vi "VISA Write and Read.vi"(6 "Delay":u32=50, 7 "Checksum":T1, 8 "error in (no error)":errorcluster, 10 "Command":string, 11 "VISA In":refnum<visa-resource-name>) -> (0 "error out":errorcluster, 2 "Response":string, 3 "VISA Out":refnum<visa-resource-name>)   [LabVIEW 2014, in "VISA.lvlib"]
uses:
  VISA.lvlib
  Checksum.ctl
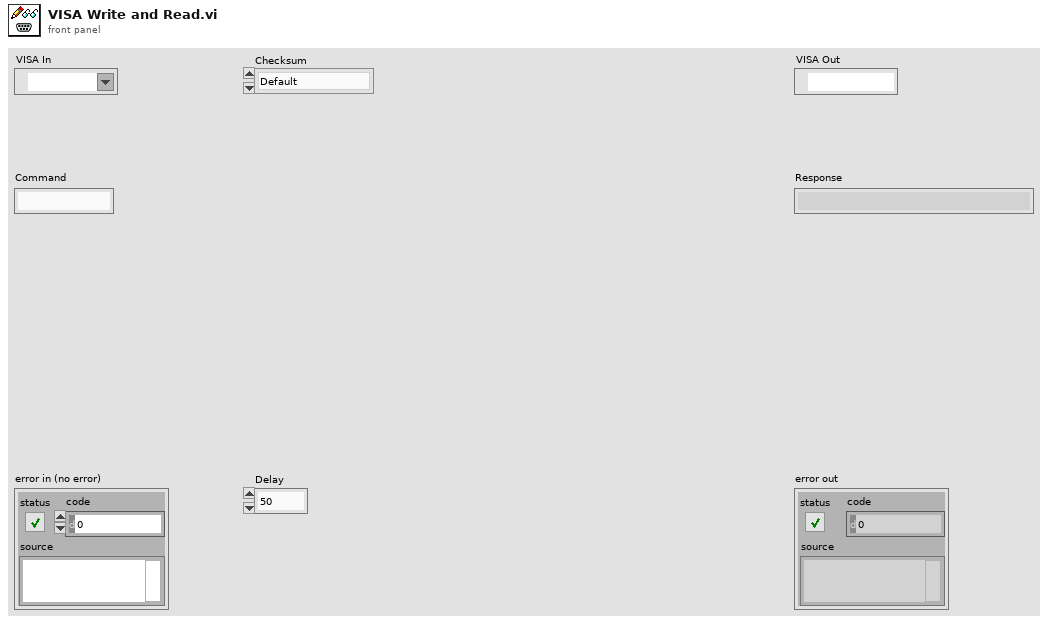
[diagram p1: front panel]
types:
  T1 = typedef "VISA.lvlib/Checksum.ctl" = enum16{"Default", "CRC"}
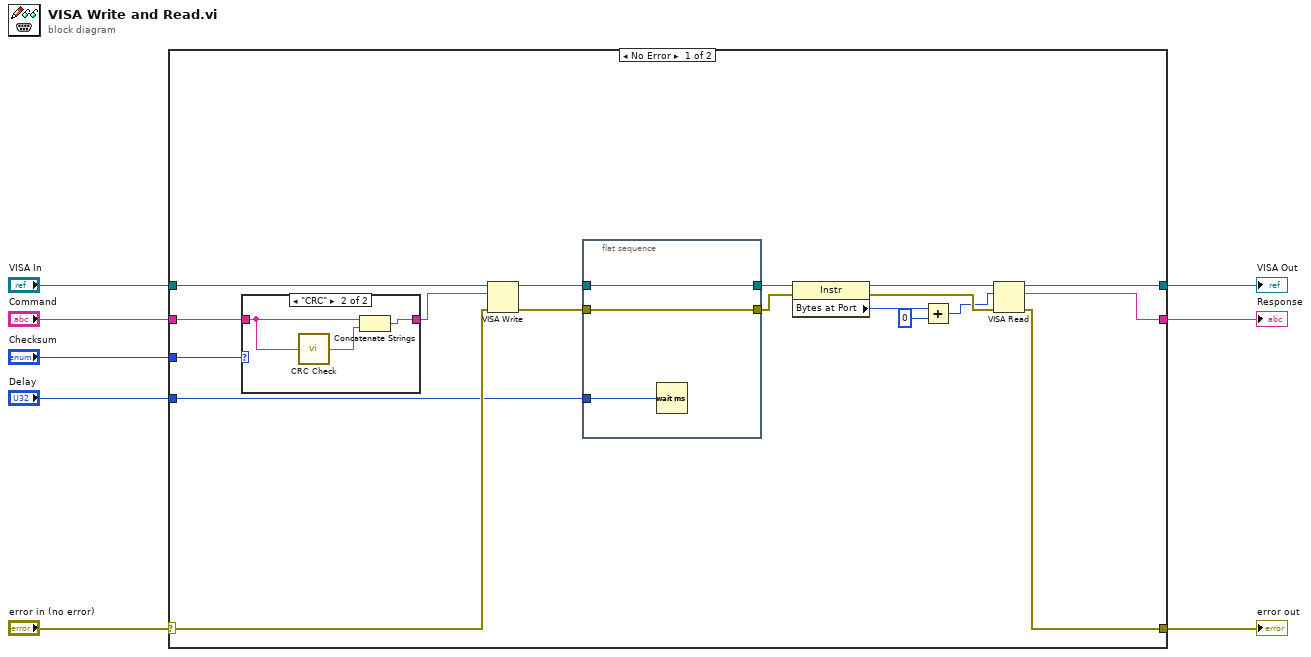
[diagram p0: block diagram]
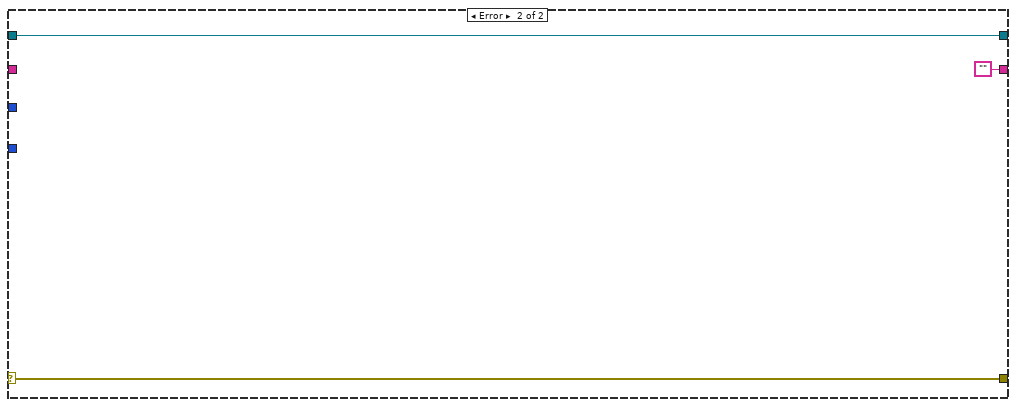
[diagram p3: hidden frame]
diagram:
  n1 = case shown="No Error" "error in (no error)" {
    selector: "error in (no error)" -> [w25 w36]
    tunnel: [w24 w36] -> w7
    tunnel: "Delay" -> [w17 _]
    tunnel: "VISA In" -> [w16 w35]
    tunnel: "Command" -> [w12 _]
    tunnel: [w15 w35] -> w3
    tunnel: [w14 "" ("read buffer")] -> w2
    tunnel: "Checksum" -> [w13 _]
    frame No Error {
      n2 = case shown="\"CRC\"" w13 {
        tunnel: w12 -> [w27 w30]
        tunnel: [w27 w29] -> w11
        frame "Default", Default {
        }
        frame "CRC" {
          n3 = call "CRC Check.vi"("Command"=w30) -> ("CRC Result"=w28:string)  [unwired: 1 out]
          n4 = Concatenate Strings(w30, w28) -> (w29:string)
        }
      }
      n5 = VISA Write(VISA resource name=w16, write buffer=w11, error in (no error)=w25) -> (VISA resource name out=w23:refnum<visa-resource-name>, error out=w26:errorcluster)  [unwired: 1 out]
      n6 = flat-sequence {
        tunnel: w26 -> [w33]
        tunnel: [w33] -> w18
        tunnel: w23 -> [w32]
        tunnel: [w32] -> w22
        tunnel: w17 -> [w31]
        frame #0 {
          n7 = Wait (ms)(milliseconds to wait=w31) -> ()  [unwired: 1 out]
        }
      }
      n8 = property class="Instr"(reference=w22, error in=w18) -> (reference out=w20:refnum<visa-resource-name>, error out=w19:errorcluster, "Bytes at Port"=w21:u32)
      n9 = Add(x=w21, y=u32 0) -> (x+y=w9:u32)
      n10 = VISA Read(VISA resource name=w20, byte count=w9, error in (no error)=w19) -> (VISA resource name out=w15:refnum<visa-resource-name>, read buffer=w14:string, error out=w24:errorcluster)  [unwired: 1 out]
    }
    frame Error {
    }
  }
  "error out" <- w7
  "VISA Out" <- w3
  "Response" <- w2
